vi "PI_GCS2_Sample_Application_PILightning.vi"() -> ()   [LabVIEW 2020]
doc: "This VI demonstrates how to use the PI GCS3 data recorder functionality. The diagram shows how to combine the driver VIs for these tasks.\n\nWarning: Before running this VI, modify the interface settings on the block diagram to reflect your configuration. The predefined settings provided with the VI probably do not match your system.\n\nCompatibility: This sample requires a PI GCS 3.0 controller."
uses:
  Low Level/Communication/Interface Settings.ctl
panel:
  out "Scan ResultID":i32[](array[numeric])
  out "Scan ResultID Meaning":string[](array[string])
  in  "Alignment input channel settings":cluster{"Alignment signal input channel":i32}={"Alignment signal input channel"=1}
  in  "Search time settings":cluster{"Maximum search time [s]":dbl}={"Maximum search time [s]"=10.0} {"Maximum search time [s]" format="%.4f"}
  in  "Threshold calculation settings":cluster{"Threshold calculation":bool}={"Threshold calculation"=TRUE}
  in  "Minimum threshold settings":cluster{"Threshold sigma":i32}={"Threshold sigma"=100}
  in  "Step axis settings":T1={"Step axis"="", "Range step axis"=100.0, "Mid. pos. step axis"=50.0, "Calc. pos. step axis"=1.0} {"Calc. pos. step axis" format="%.4f"; "Mid. pos. step axis" format="%.4f"; "Range step axis" format="%.4f"}
  in  "Scan axis settings":T2={"Scan axis"="", "Range scan axis"=100.0, "Mid. pos. scan axis"=50.0, "Calc. pos. scan axis"=1.0} {"Calc. pos. scan axis" format="%.4f"; "Mid. pos. scan axis" format="%.4f"; "Range scan axis" format="%.4f"}
  in  "Position before Scan":dbl[](array[numeric]) format="%.6f"
  out "Conn. Axes":string[](array[string])
  out "Identification":string
  out "error out":errorcluster
  in  "error in (no error)":errorcluster
  # "This VI demonstrates how to use PILightning.\nThe diagram shows how to combine the driver VIs for these tasks. \n\nWarning: Before running this VI, modify the interface settings on the block diagram to reflect your configuration.\n                 The predefined settings provided with the VI probably do not match your system.\n\nCompatibility: This sample requires a PI GCS 2.0 controller with support for the GCS command FDL."
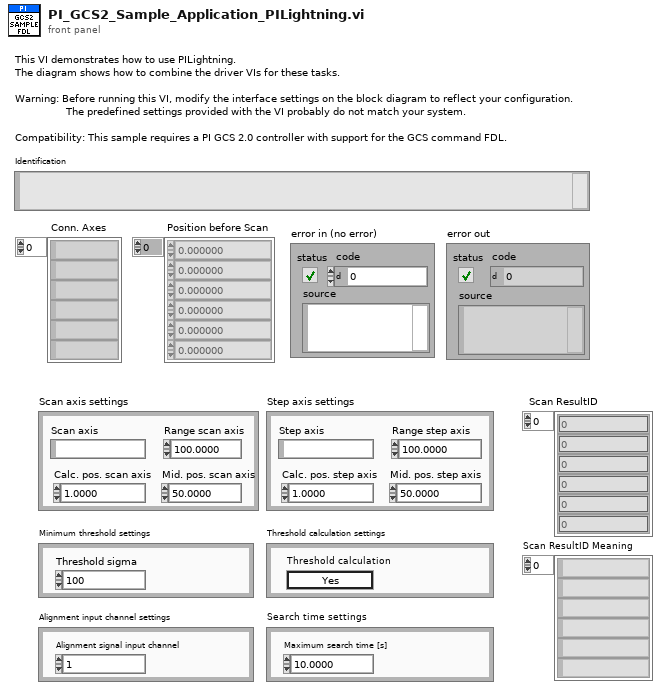
[diagram p1: front panel]
types:
  T1 = cluster{"Step axis":string, "Range step axis":dbl, "Mid. pos. step axis":dbl, "Calc. pos. step axis":dbl}
  T2 = cluster{"Scan axis":string, "Range scan axis":dbl, "Mid. pos. scan axis":dbl, "Calc. pos. scan axis":dbl}
  T3 = enum16{"Do not reference", "Reference switch", "Negative limit switch", "Positive limit switch"}[]
  T4 = typedef "Interface Settings.ctl" = cluster{"Interface":u16, "Timeout":u32, "RS232 settings":cluster{"Portnumber":u8, "Baudrate":u16}, "TCP/IP settings":cluster{"Host address/name":string, "Port":i32, "Board":i32, "TCP/IP Search?":bool}, "USB settings":cluster{"S/N":string, "USB Search?":bool}, "DaisyChain settings":cluster{"Register DC":bool, "DaisyChain Search?":bool, "Device ID":i32}, "DLL for Device":u16}
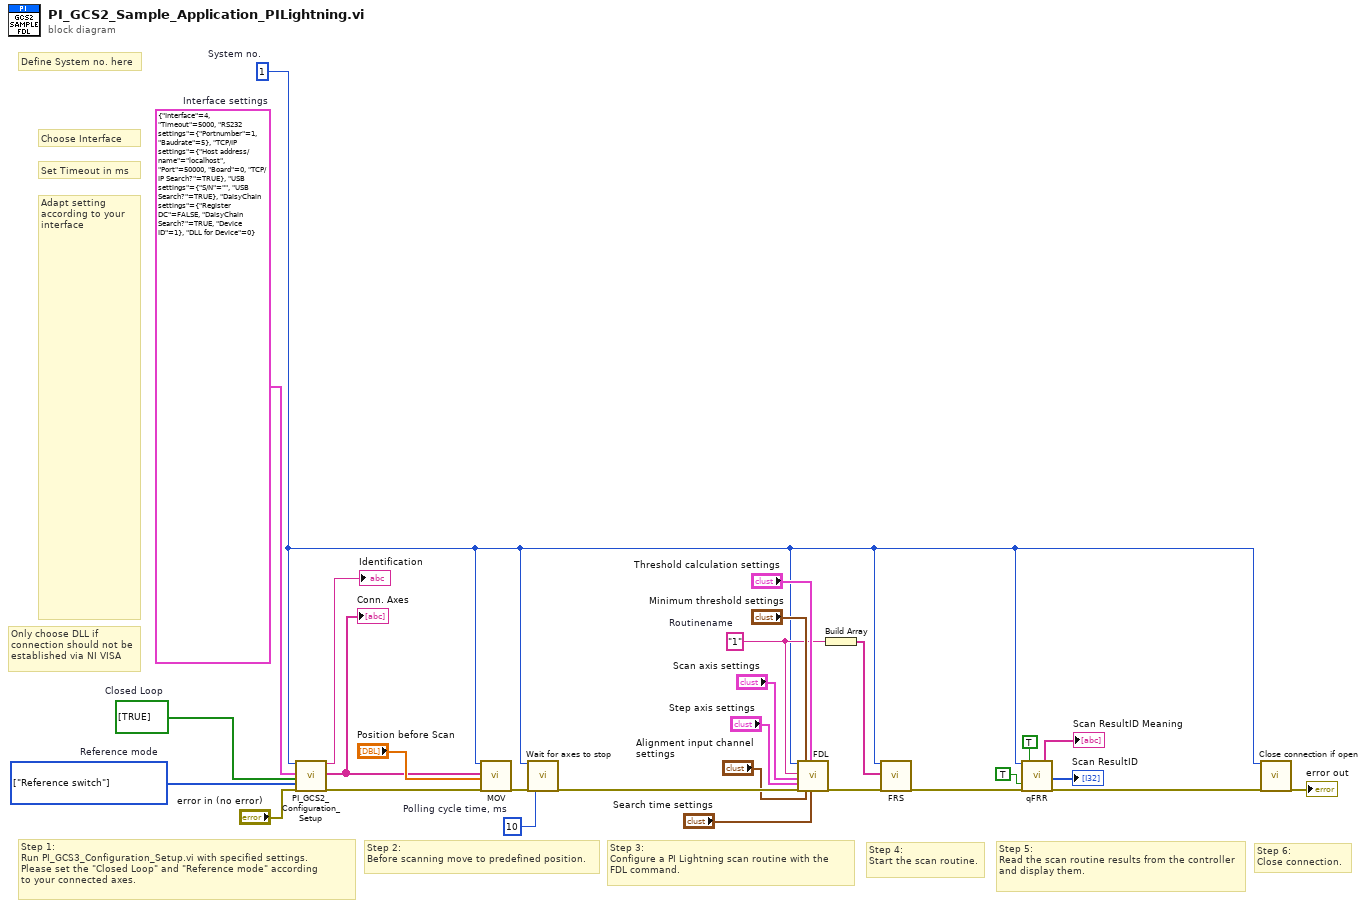
[diagram p0: block diagram]
diagram:
  w10 = "1"  # Routinename
  w22 = u32 10  # Polling cycle time, ms
  w23 = T3 [enum."Reference switch"] items=["Do not reference", "Reference switch", "Negative limit switch", "Positive limit switch"]  # Reference mode
  w24 = bool[] [TRUE]  # Closed Loop
  w25 = T4 {"Interface"=4, "Timeout"=5000, "RS232 settings"={"Portnumber"=1, "Baudrate"=5}, "TCP/IP settings"={"Host address/name"="localhost", "Port"=50000, "Board"=0, "TCP/IP Search?"=TRUE}, "USB settings"={"S/N"="", "USB Search?"=TRUE}, "DaisyChain settings"={"Register DC"=FALSE, "DaisyChain Search?"=TRUE, "Device ID"=1}, "DLL for Device"=0}  # Interface settings
  w6 = 1  # System no.
  # "Define System no. here"
  # "Adapt setting according to your interface"
  # "Set Timeout in ms"
  # "Choose Interface"
  # "Only choose DLL if connection should not be established via NI VISA"
  # "Step 4:\nStart the scan routine."
  # "Step 5:\nRead the scan routine results from the controller\nand display them."
  # "Step 3:\nConfigure a PI Lightning scan routine with the\nFDL command."
  # "Step 2:\nBefore scanning move to predefined position."
  # "Step 6:\nClose connection."
  # "Step 1:\nRun PI_GCS3_Configuration_Setup.vi with specified settings.\nPlease set the \"Closed Loop\" and \"Reference mode\" according\nto your connected axes."
  n1 = call "PI_GCS2_Configuration_Setup.vi"("System no."=w6, "Interface settings"=w25, "Closed Loop"=w24, "Reference mode"=w23, "error in"="error in (no error)") -> ("Identification"=→"Identification":string, "Conn. Axis"=w19:string[], "error out"=w21:errorcluster)  [unwired: 9 in, 3 out]
  "Conn. Axes" <- w19
  n2 = call "MOV.vi"("System no."=w6, "Axes to move"=w19, "Position values"="Position before Scan", "error in"=w21) -> ("error out"=w18:errorcluster)  [unwired: 15 in]
  n3 = call "Wait for axes to stop.vi"("System no."=w6, "error in"=w18, "Polling cycle time, ms"=w22) -> ("error out"=w17:errorcluster)  [unwired: 15 in, 1 out]
  n4 = call "FDL.vi"("System no."=w6, "Routinename"=w10, "Scan axis settings"="Scan axis settings", "Step axis settings"="Step axis settings", "error in"=w17, "Minimum threshold settings"="Minimum threshold settings", "Alignment input channel settings"="Alignment input channel settings", "Threshold calculation settings"="Threshold calculation settings", "Search time settings"="Search time settings") -> ("error out"=w9:errorcluster)  [unwired: 10 in]
  n5 = Build Array(w10) -> (w5:string[])
  n6 = call "FRS.vi"("System no."=w6, "Routines to start"=w5, "error in"=w9) -> ("error out"=w7:errorcluster)  [unwired: 16 in]
  n7 = call "qFRR.vi"("System no."=w6, "Query all?"=TRUE, "error in"=w7, "Use FRH?"=TRUE) -> ("ResultID Meaning"=→"Scan ResultID Meaning":string[], "ResultID out"=→"Scan ResultID":i32[], "error out"=w8:errorcluster)  [unwired: 9 in, 4 out]
  n8 = call "Close connection if open.vi"("System no."=w6, "error in"=w8) -> ("error out"=→"error out":errorcluster)  [unwired: 16 in, 1 out]
